vi "Tone-Glide.vi"(0 "New":T1, 5 "Old":T1, 7 "Fs (Hz)":dbl=100000.0, 9 "Npts":i32, 12 "Original method?":bool=TRUE) -> (4 "Params out":T1, 8 "Y":dbl[](array[numeric]))   [LabVIEW 2015]
uses:
  Tone Params.ctl
  <vilib>/Analysis/1siggen.llb/Ramp Pattern by Samples.vi
  <vilib>/Analysis/NI_AALBase.lvlib
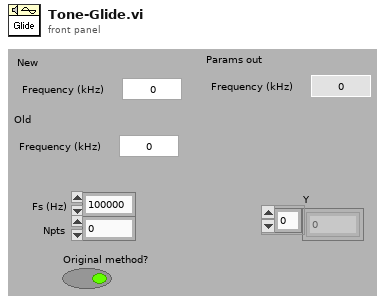
[diagram p1: front panel]
types:
  T1 = typedef "Tone Params.ctl" = cluster{"Frequency (kHz)":dbl, "Last Freq":dbl, "Last Phase":dbl}
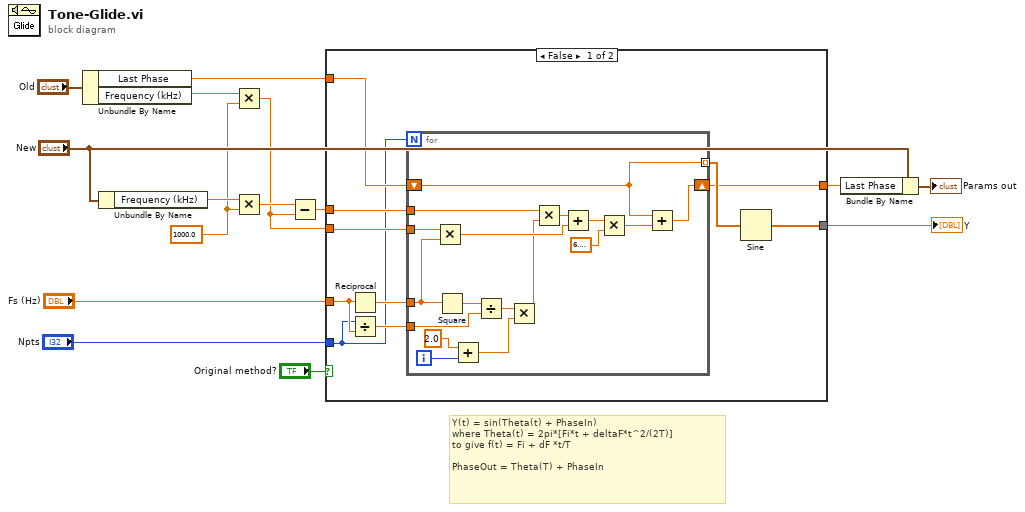
[diagram p0: block diagram]
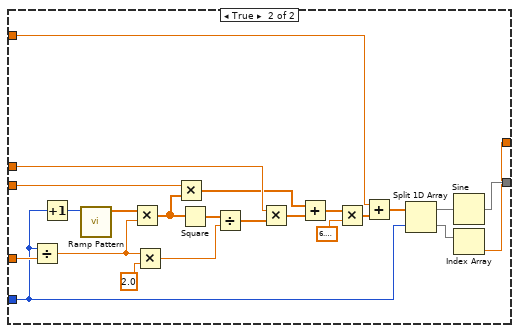
[diagram p2: hidden frame]
diagram:
  w2 = 1000.0 ("y")
  # "Y(t) = sin(Theta(t) + PhaseIn)\nwhere Theta(t) = 2pi*[Fi*t + deltaF*t^2/(2T)]\nto give f(t) = Fi + dF *t/T \n\nPhaseOut = Theta(T) + PhaseIn"
  n1 = Unbundle By Name("Old") -> ("Last Phase"=w5:dbl, "Frequency (kHz)"=w4:dbl)
  n2 = Unbundle By Name("New") -> ("Frequency (kHz)"=w11:dbl)
  n3 = Multiply(x=w4, y=w2) -> (x*y=w3:dbl)
  n4 = Multiply(x=w11, y=w2) -> (x*y=w8:dbl)
  n5 = Subtract(x=w8, y=w3) -> (x-y=w12:dbl)
  n6 = case shown="False" "Original method?" {
    tunnel: "Fs (Hz)" -> [w17 w65]
    tunnel: "Npts" -> [w16 w64]
    tunnel: [w18 w63] -> w13
    tunnel: w12 -> [w21 w62]
    tunnel: [w19 w61] -> w9
    tunnel: w5 -> [w22 w60]
    tunnel: w3 -> [w20 w59]
    frame False {
      n7 = Reciprocal(x=w17) -> (1/x=w25:dbl)
      n8 = Divide(x=w16, y=w17) -> (x/y=w24:dbl)
      n9 = for {
        N: w16 -> [_]
        tunnel: w25 -> [w41]
        shift-right: [w33] -> w19
        shift-left: w22 -> [w32]
        tunnel: w20 -> [w42]
        tunnel: w24 -> [w30]
        tunnel: w21 -> [w31]
        tunnel: [w32] -> w23 mode=indexing
        i -> [w28]
        n10 = Multiply(x=w42, y=w41) -> (x*y=w37:dbl)
        n11 = Square(x=w41) -> (x^2=w40:dbl)
        n12 = Add(x=2.0, y=w28) -> (x+y=w26:dbl)
        n13 = Divide(x=w40, y=w30) -> (x/y=w39:dbl)
        n14 = Multiply(x=w39, y=w26) -> (x*y=w29:dbl)
        n15 = Multiply(x=w31, y=w29) -> (x*y=w38:dbl)
        n16 = Add(x=w38, y=w37) -> (x+y=w36:dbl)
        n17 = Multiply(x=w36, y=6.283185307179586) -> (x*y=w34:dbl)
        n18 = Add(x=w32, y=w34) -> (x+y=w33:dbl)
      }
      n19 = Sine(x=w23) -> (sin(x)=w18:dbl[])
    }
    frame True {
      n20 = Divide(x=w64, y=w65) -> (x/y=w50:dbl)
      n21 = Increment(x=w64) -> (x+1=w46:i32)
      n22 = call-poly <vilib>:"Ramp Pattern.vi"("samples"=w46) -> ("Ramp Pattern"=w58:dbl[])  [unwired: 9 in, 1 out]
      n23 = Multiply(x=w58, y=w50) -> (x*y=w49:dbl[])
      n24 = Multiply(x=w50, y=2.0) -> (x*y=w55:dbl)
      n25 = Multiply(x=w59, y=w49) -> (x*y=w47:dbl[])
      n26 = Square(x=w49) -> (x^2=w56:dbl[])
      n27 = Divide(x=w56, y=w55) -> (x/y=w54:dbl[])
      n28 = Multiply(x=w62, y=w54) -> (x*y=w53:dbl[])
      n29 = Add(x=w47, y=w53) -> (x+y=w48:dbl[])
      n30 = Multiply(x=w48, y=6.283185307179586) -> (x*y=w51:dbl[])
      n31 = Add(x=w60, y=w51) -> (x+y=w45:dbl[])
      n32 = Split 1D Array(array=w45, index=w64) -> (first subarray=w44:dbl[], second subarray=w43:dbl[])
      n33 = Sine(x=w44) -> (sin(x)=w63:dbl[])
      n34 = Index Array(array=w43) -> (element=w61:dbl)  [unwired: 1 in]
    }
  }
  "Y" <- w13
  n35 = Bundle By Name(cluster="New", "Last Phase"=w9) -> (→"Params out":T1)
